vi "8164B SendStringToSlot.vi"(8 "error in":errorcluster, 9 "Slot Number":i32, 10 "CMD":string, 11 "KeySight 8164B control in":T1) -> (0 "error out":errorcluster, 3 "KeySight 8164B control out":T1)   [LabVIEW 2018, in "KeySight 8164B LAN InstrLib.lvlib"]
uses:
  KeySight 8164B LAN InstrLib.lvlib
  typedefs/KeySight 8164B control.ctl
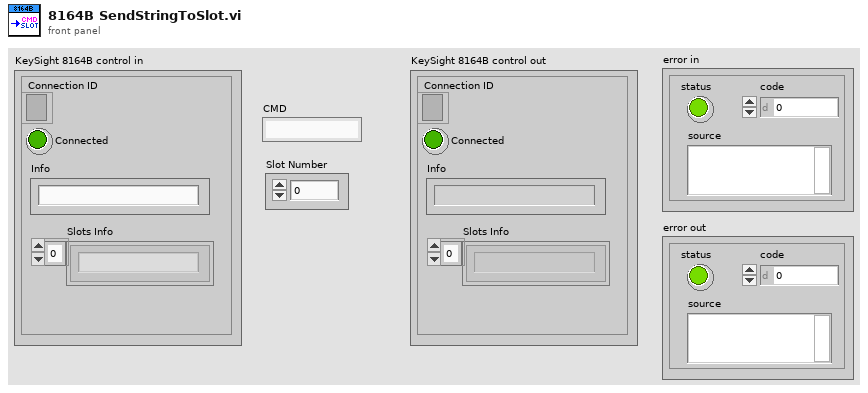
[diagram p1: front panel]
types:
  T1 = typedef "KeySight 8164B LAN InstrLib.lvlib/KeySight 8164B control.ctl" = cluster{"Connection ID":refnum<k5>, "Connected":bool, "Info":string, "Slots Info":string[]}
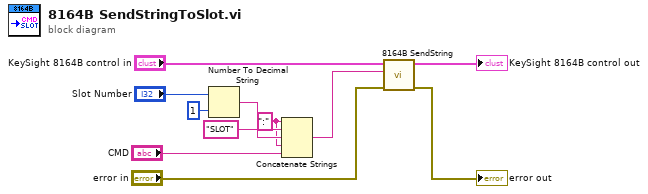
[diagram p0: block diagram]
diagram:
  w5 = ":" ("string")
  n1 = Number To Decimal String(number="Slot Number", width (-)=i16 1) -> (decimal integer string=w6:string)
  n2 = Concatenate Strings(w5, "SLOT", w6, w5, "CMD") -> (w3:string)
  n3 = call "8164B SendString.vi"("error in"="error in", "CMD"=w3, "KeySight 8164B control in"="KeySight 8164B control in") -> ("error out"=→"error out":errorcluster, "KeySight 8164B control out"=→"KeySight 8164B control out":T1)  [unwired: 7 in]
